vi "Write and Read Multiple Registers Response.vi"(8 "error in (no error)":errorcluster, 9 "Modbus Data Unit in":T1={"function"=1, "Data"=[]} {"function" items=["Read Discrete Inputs"=2, "Read Coils"=1, "Write Single Coil"=5, "Write Multiple Coils"=15, "Read Input Register"=4, "Read Holding Registers"=3, "Write Single Register"=6, "Write Multiple Registers"=16, "Read/Write Multiple Registers"=23, "Mask Write Register"=22, "Read FIFO Queue"=24, "Read File Record"=20, "Write File Record"=21, "Read Exception Status"=7, "Diagnostic"=8, "Get Com Event Counter"=11, "Get Com Event Log"=12, "Report Slave ID"=17, "Read Device Identification"=43]; "Data" format="%.0x"}) -> (0 "error out":errorcluster, 1 "registers":u16[](array[numeric]), 2 "byte count":u8)   [LabVIEW 2019, in "NI_modbus_upd.lvlib"]
doc: "Decodes the response generated by the write and read multiple holding registers function."
uses:
  NI_modbus_upd.lvlib
  Ctl/MB Modbus Data Unit.ctl
  Modbus Data Unit (PDU)/Function.ctl
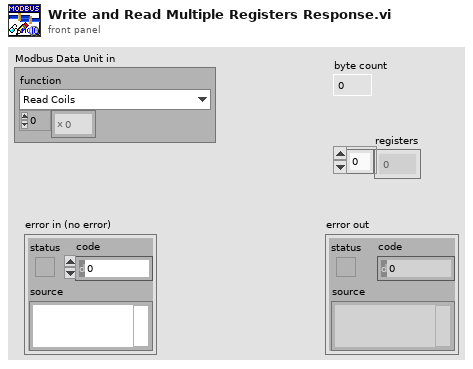
[diagram p1: front panel]
types:
  T1 = typedef "NI_modbus_upd.lvlib/MB Modbus Data Unit.ctl" = cluster{"function":T2, "Data":u8[]}
  T2 = typedef "NI_modbus_upd.lvlib/Function.ctl" = u8
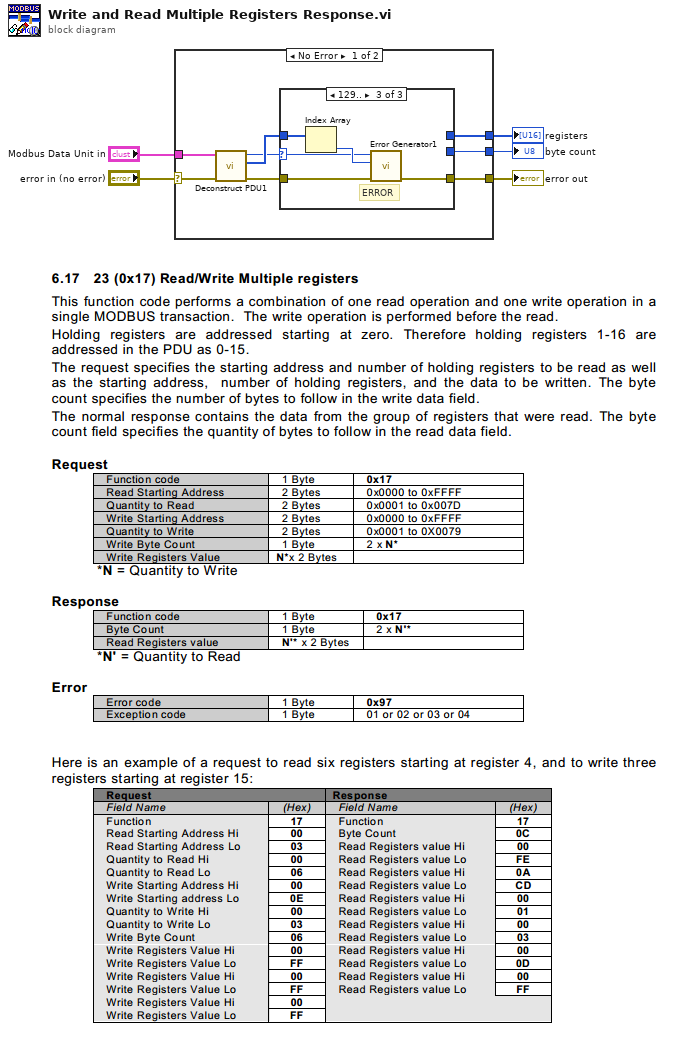
[diagram p0: block diagram]
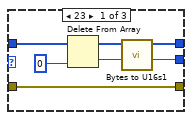
[diagram p2: hidden frame]
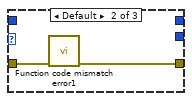
[diagram p3: hidden frame]
diagram:
  n1 = case shown="No Error" "error in (no error)" {
    selector: "error in (no error)" -> [w12 w27]
    tunnel: [w13 w27] -> w4
    tunnel: "Modbus Data Unit in" -> [w6 _]
    tunnel: [w8 _] -> w3
    tunnel: [w7 _] -> w2
    frame No Error {
      n2 = call "Deconstruct PDU1.vi"("error in (no error)"=w12, "Modbus Data Unit in"=w6) -> ("error out"=w10:errorcluster, "data"=w11:u8[], "function"=w9:T2)  [unwired: 7 in]
      n3 = case shown="129.." w9 {
        selector: w9 -> [_ _ w22]
        tunnel: w10 -> [w19 w21 w23]
        tunnel: w11 -> [w16 _ w26]
        tunnel: [w19 w20 w25] -> w13
        tunnel: [w15 _ _] -> w8
        tunnel: [w14 _ _] -> w7
        frame 23 {
          n4 = Delete From Array(array=w16, index=0) -> (deleted portion=w15:u8, array with subset deleted=w17:u8[])  [unwired: 1 in]
          n5 = call "Bytes to U16s1.vi"("bytes"=w17) -> ("registers"=w14:u16[])  [unwired: 10 in]
        }
        frame Default {
          n6 = call "Function code mismatch error1.vi"("error in (no error)"=w21) -> ("error out"=w20:errorcluster)  [unwired: 10 in]
        }
        frame 129.. {
          # "ERROR"
          n7 = Index Array(array=w26) -> (element=w24:u8)  [unwired: 1 in]
          n8 = call "Error Generator1.vi"("error in (no error)"=w23, "data return (error code)"=w24, "function return"=w22) -> ("error out"=w25:errorcluster)  [unwired: 8 in]
        }
      }
    }
    frame Error {
    }
  }
  "error out" <- w4
  "byte count" <- w3
  "registers" <- w2
